vi "Global Stop Actions.vi"(8 "error in (no error)":errorcluster, 9 "Stop on Error?":bool, 10 "Stop?":bool, 11 "Stop Ref":refnum<data-value>) -> (0 "error out":errorcluster {"code" min=0 max=0}, 2 "Latched Stop":bool, 3 "Stop Ref":refnum<data-value>)   [LabVIEW 2015, in "OPC UA Client Engine.lvlib"]
uses:
  OPC UA Client Engine.lvlib
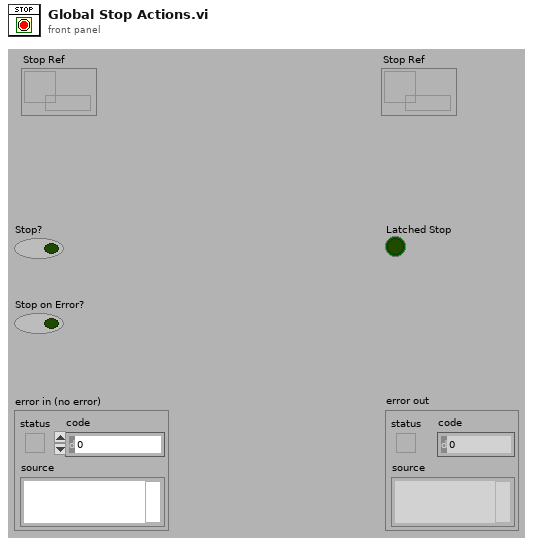
[diagram p1: front panel]
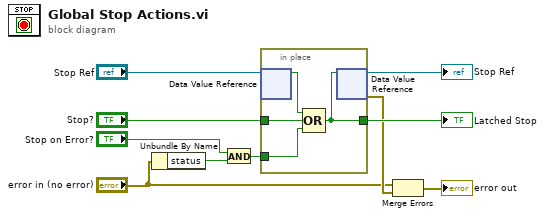
[diagram p0: block diagram]
diagram:
  n1 = Unbundle By Name("error in (no error)") -> ("status"=w9:bool)
  n2 = And(x="Stop on Error?", y=w9) -> (x .and. y?=w8:bool)
  n3 = in-place {
    in-place-border: [w12] -> w4
    in-place-border: w8 -> [w13]
    in-place-border: "Stop?" -> [w11]
    n4 = in-place-dvr #1("Stop Ref") -> (w14:bool)  [unwired: 1 out]
    n5 = Compound Arithmetic op=OR(w14, w11, w13) -> (w12:bool)
    n6 = in-place-dvr #1(w12) -> (→"Stop Ref":refnum<data-value>, w2:errorcluster)
  }
  "Latched Stop" <- w4
  n7 = Merge Errors("error in (no error)", w2) -> (→"error out":errorcluster)
